vi "Create.vi"(8 "error in (no error)":errorcluster, 11 "State type":refnum<class "State.lvclass">) -> (0 "error out":errorcluster, 3 "State out":refnum<class "State.lvclass">)   [LabVIEW 2019, in "DSF Core.lvlib" / "State.lvclass"]
uses:
  State.lvclass
  State Data.ctl
  State.lvclass/State.ctl
  <vilib>/NI/Memory Manager/Classes/Pointer/Pointer.lvclass/Pointer.ctl
  <vilib>/NI/Memory Manager/Classes/Pointer/Set Address.vi
  <vilib>/NI/Memory Manager/Classes/Pointer/Set Size.vi
  <vilib>/NI/Memory Manager/Classes/Pointer/Set Internal.vi
  <vilib>/NI/Memory Manager/Classes/Pointer/Pointer.lvclass
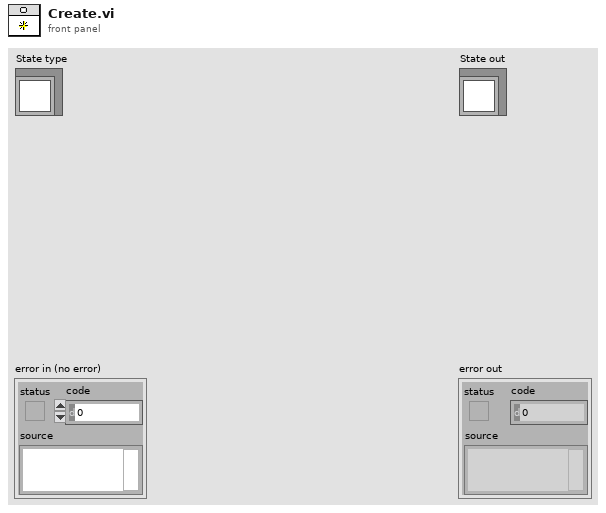
[diagram p1: front panel]
types:
  T1 = typedef "DSF Core.lvlib/State.lvclass/State Data.ctl" = cluster{"state":u8}
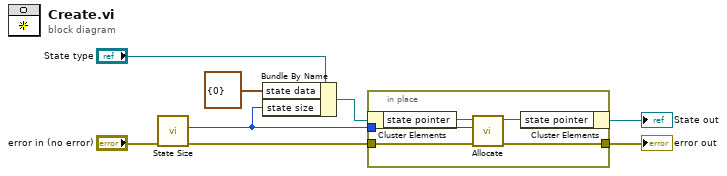
[diagram p0: block diagram]
diagram:
  n1 = call "State Size.vi"("error in (no error)"="error in (no error)") -> ("error out"=w5:errorcluster, "size"=w3:u64)  [unwired: 9 in]
  n2 = Bundle By Name(cluster="State type", "state data"=T1 {"state"=0}, "state size"=w3) -> (w1:refnum<class "State.lvclass">)
  n3 = in-place {
    in-place-border: [w13] -> w8
    in-place-border: w5 -> [w10]
    in-place-border: w3 -> [w11]
    n4 = in-place-cluster #1(w1) -> ("state pointer"=w9:refnum<class "Pointer.lvclass">)
    n5 = call <vilib>:"Allocate.vi"("error in (no error)"=w10, "size"=w11, "Pointer type"=w9) -> ("error out"=w13:errorcluster, "Pointer out"=w12:refnum<class "Pointer.lvclass">)  [unwired: 7 in]
    n6 = in-place-cluster #1("state pointer"=w12) -> (→"State out":refnum<class "State.lvclass">)
  }
  "error out" <- w8
